vi "nifxpmath_DiscreteDelay_ArrayTemplate.vi"(1 "init on first call":bool, 2 "n-1":u16, 3 "enable":bool=TRUE, 4 "D":bool[](array[boolean])) -> (0 "Q":bool[](array[boolean]))   [LabVIEW 2017]
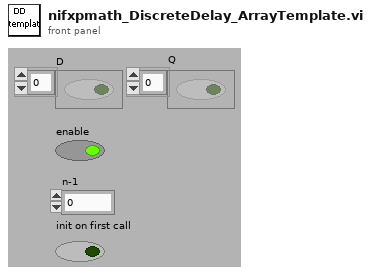
[diagram p1: front panel]
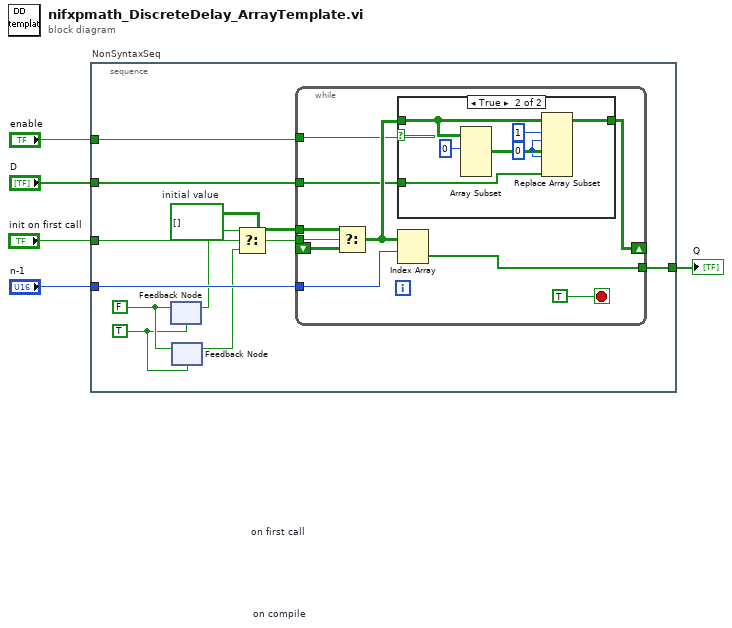
[diagram p0: block diagram]
diagram:
  n1 = stacked-sequence "NonSyntaxSeq" {
    tunnel: "enable" -> [w16]
    tunnel: "D" -> [w15]
    tunnel: "n-1" -> [w14]
    tunnel: [w13] -> w2
    tunnel: "init on first call" -> [w8]
    frame #0 {
      w6 = bool[][] []  # initial value
      w11 = TRUE
      w12 = FALSE
      n2 = feedback-in #1(w12) -> ()
      n3 = feedback #1 "on first call"(w11) -> (w10:bool)
      n4 = feedback-in #2(w12) -> ()
      n5 = feedback #2 "on compile"(w11) -> (w9:bool)
      n6 = Select(t=w10, s=w8, f=w9) -> (s? t:f=w7:bool)
      n7 = while {
        shift-right: [w24] -> _
        shift-left: _ -> [w18]
        tunnel: w6 -> [w19]
        tunnel: w15 -> [w23]
        tunnel: [w22] -> w13
        tunnel: w16 -> [w21]
        tunnel: w14 -> [w20]
        tunnel: w7 -> [w17]
        stop <- TRUE stop-if-true
        n8 = Select(t=w19, s=w17, f=w18) -> (s? t:f=w25:bool[][])
        n9 = case shown="True" w21 {
          tunnel: w23 -> [_ w29]
          tunnel: w25 -> [w27 w33]
          tunnel: [w27 w28] -> w24
          frame False {
          }
          frame True {
            w30 = 0 ("disabled index (col)")
            n10 = Array Subset(array=w33, index (row)=0 ("index")) -> (w31:bool[][])  [unwired: 3 in]
            n11 = Replace Array Subset(array=w33, new element #1=w31, index (row) #1=1 ("index (row)"), index (col) #1=w30, new element #2=w29, index (row) #2=w30) -> (w28:bool[][])  [unwired: 1 in]
          }
        }
        n12 = Index Array(array=w25, index (row)=w20) -> (element=w22:bool[])  [unwired: 1 in]
      }
    }
  }
  "Q" <- w2
